vi "Constants.vi"() -> ()   [LabVIEW 2015, in "PXIe 4113 Shared.lvlib"]
doc: "Use this Global VI to access the GUIDs assigned to the page resources of the Custom Device."
uses:
  PXIe 4113 Shared.lvlib
panel:
  in  "Tab Control":enum32{"GUIDS", "Constants", "Properties"}(tab)
  in  "PXIe 4113":string="6263214c-13bb-47a3-9793-857264327de1"
  in  "Hardware Device Name":string="Hardware Device Name"
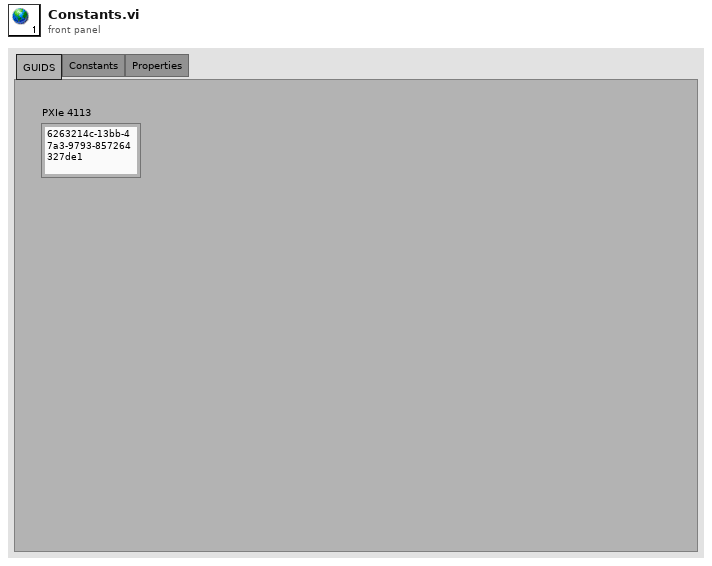
[diagram p1: front panel]
diagram:
